vi "Set Property.vi"(10 "Ctl Ref":refnum<vi>, 11 "CaptionUIP In":refnum<class "CaptionUIP.lvclass">) -> (0 "Error Out":errorcluster, 3 "CaptionUIP Out":refnum<class "CaptionUIP.lvclass">)   [LabVIEW 2020, in "UIM.lvlib" / "CaptionUIP.lvclass"]
doc: "Modify this method to implement functionality for applying the UIP data to the property from VI Server Control."
uses:
  CaptionUIP.lvclass
  CaptionUIP.lvclass/CaptionUIP.ctl
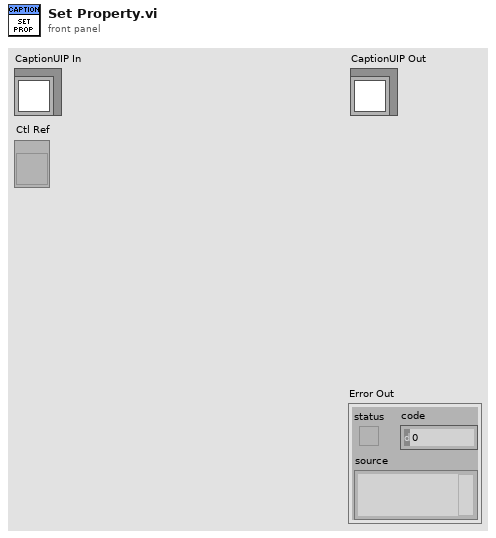
[diagram p1: front panel]
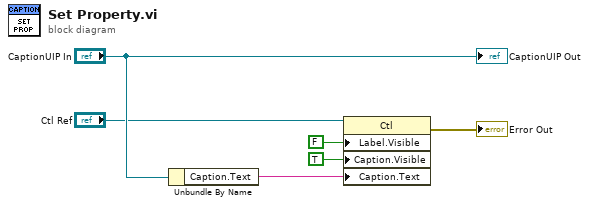
[diagram p0: block diagram]
diagram:
  n1 = Unbundle By Name("CaptionUIP In") -> ("Caption.Text"=w4:string)
  n2 = property class="Ctl"(reference="Ctl Ref", "Label.Visible"=FALSE, "Caption.Visible"=TRUE, "Caption.Text"=w4) -> (error out=→"Error Out":errorcluster)  [unwired: 1 in, 1 out]
  "CaptionUIP Out" <- "CaptionUIP In"
